vi "DUAL GAUGE-Convert2Eng.vi"(7 "W/R [W: Int in; Str out ]":bool, 8 "Kommastellen":u8=2, 9 "Eng2 in":dbl format="%.2e", 10 "Eng1 in":dbl format="%.2e", 11 "String in":string) -> (1 "Eng2 out":dbl format="%.2e", 2 "Eng1 out":dbl format="%.2e", 3 "String out":string)   [LabVIEW 2010, in "Dual Gauge.lvlib"]
uses:
  Dual Gauge.lvlib
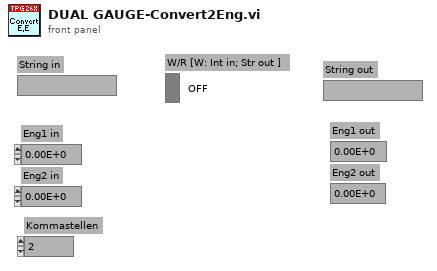
[diagram p1: front panel]
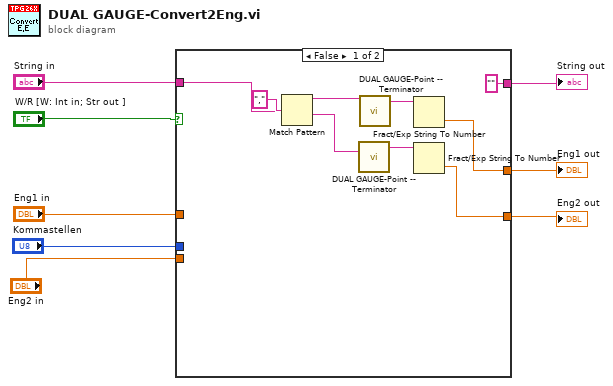
[diagram p0: block diagram]
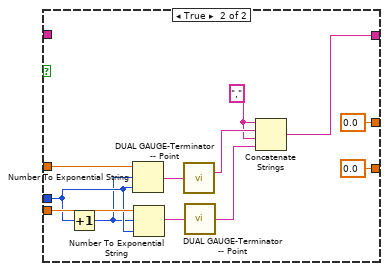
[diagram p2: hidden frame]
diagram:
  n1 = case shown="False" "W/R [W: Int in; Str out ]" {
    tunnel: "Eng1 in" -> [_ w29]
    tunnel: "Eng2 in" -> [_ w28]
    tunnel: ["" w23] -> w5
    tunnel: "String in" -> [w16 _]
    tunnel: [w13 0.0] -> w3
    tunnel: [w12 0.0] -> w2
    tunnel: "Kommastellen" -> [_ w19]
    frame False {
      n2 = Match Pattern(string=w16, regular expression=",") -> (before substring=w10:string, after substring=w9:string)  [unwired: 1 in, 2 out]
      n3 = call "DUAL GAUGE-Point -- Terminator.vi"("Eingangstring"=w9) -> ("Ausgangstring"=w14:string)
      n4 = call "DUAL GAUGE-Point -- Terminator.vi"("Eingangstring"=w10) -> ("Ausgangstring"=w15:string)
      n5 = Fract/Exp String To Number(string=w15) -> (number=w12:dbl)  [unwired: 3 in, 1 out]
      n6 = Fract/Exp String To Number(string=w14) -> (number=w13:dbl)  [unwired: 3 in, 1 out]
    }
    frame True {
      w20 = ","
      n7 = Increment(x=w19) -> (x+1=w18:u8)
      n8 = Number To Exponential String(number=w29, precision (6)=w19, 3:w18) -> (E-format string=w27:string)  [unwired: 1 in]
      n9 = Number To Exponential String(number=w28, precision (6)=w19, 3:w18) -> (E-format string=w26:string)  [unwired: 1 in]
      n10 = call "DUAL GAUGE-Terminator -- Point.vi"("Eingangstring"=w27) -> ("Ausgangstring"=w25:string)
      n11 = call "DUAL GAUGE-Terminator -- Point.vi"("Eingangstring"=w26) -> ("Ausgangstring"=w24:string)
      n12 = Concatenate Strings(w20, w25, w20, w24) -> (w23:string)
    }
  }
  "String out" <- w5
  "Eng1 out" <- w2
  "Eng2 out" <- w3
